vi "poly_persist_controls_auto_read.vi"(8 "error in":errorcluster, 10 "ctrl refs in":refnum<vi>[](array[refnum])) -> (0 "error out":errorcluster, 2 "ctrl refs out":refnum<vi>[](array[refnum]))   [LabVIEW 2015, in "_persist_controls_polys.lvlib"]
doc: "Writes the values of an array of controls to a configuration file or reads them back.\n<b>Control References</b> is an array of the references of the controls to be saved.\n\nThe configuration file is named after the VI the first control in the array is in and is saved in the LabVIEW Data folder"
uses:
  _persist_controls_polys.lvlib
  RWC_Actions.ctl
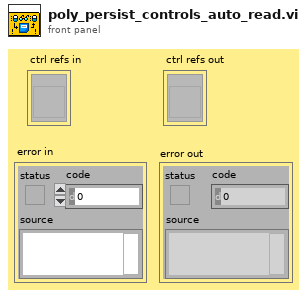
[diagram p1: front panel]
types:
  T1 = typedef "RWC_Actions.ctl" = enum16{"Read", "Write", "Read and Create"}
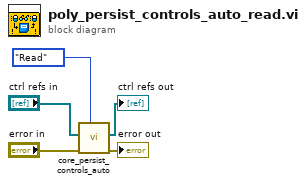
[diagram p0: block diagram]
diagram:
  n1 = call "core_persist_controls_auto.vi"("action"=RWC_Actions."Read" ("Action"), "error in"="error in", "crtl refs in"="ctrl refs in") -> ("error out"=→"error out":errorcluster, "ctrl refs out"=→"ctrl refs out":refnum<vi>[])  [unwired: 7 in]
